vi "Lockin Digitizer Output Signal.vi"(6 "decimating factor":i32=1, 8 "error in":errorcluster, 9 "Phase in":dbl format="%0.2f", 10 "Frequency":dbl=0.0078125 format="%0.4e", 11 "Input data":dbl[][](array[numeric])) -> (0 "error out":errorcluster, 1 "Phase out":dbl format="%0.2e", 2 "Y":dbl[][](array[numeric]), 3 "X":dbl[][](array[numeric]))   [LabVIEW 2021]
uses:
  <vilib>/Analysis/2dsp.llb/Decimate (single shot, DBL).vi
  <vilib>/Analysis/NI_AALBase.lvlib
  <vilib>/Analysis/NI_AALPro.lvlib
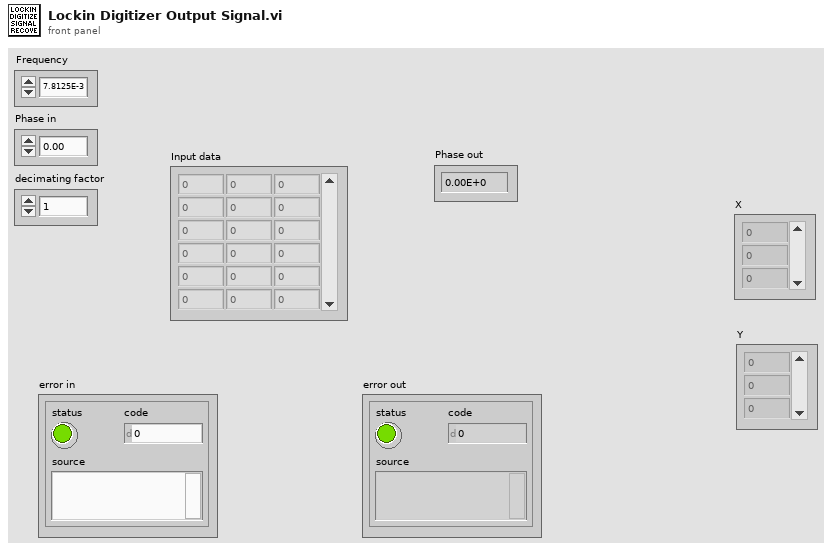
[diagram p1: front panel]
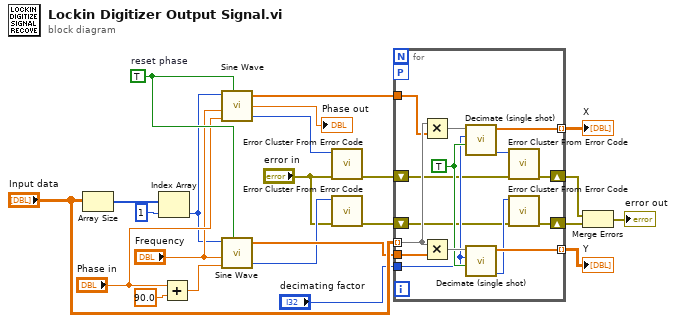
[diagram p0: block diagram]
diagram:
  w17 = TRUE  # reset phase
  n1 = Array Size(array="Input data") -> (size(s)=w23:i32[])
  n2 = Index Array(array=w23, index=1) -> (element=w12:i32)
  n3 = Add(x="Phase in", y=90.0 ("phase in")) -> (x+y=w14:dbl)
  n4 = call <vilib>:"Sine Wave.vi"("samples"=w12, "frequency"="Frequency", "phase in"="Phase in", "reset phase"=w17) -> ("sine wave"=w18:dbl[], "phase out"=→"Phase out":dbl, "error"=w20:i32)  [unwired: 1 in]
  n5 = call <vilib>:"Sine Wave.vi"("samples"=w12, "frequency"="Frequency", "phase in"=w14, "reset phase"=w17) -> ("sine wave"=w11:dbl[], "error"=w9:i32)  [unwired: 1 in, 1 out]
  n6 = call <vilib>:"Error Cluster From Error Code.vi"("error in (no error)"="error in", "error code (0)"=w20) -> ("error out"=w8:errorcluster)  [unwired: 7 in]
  n7 = call <vilib>:"Error Cluster From Error Code.vi"("error in (no error)"="error in", "error code (0)"=w9) -> ("error out"=w7:errorcluster)  [unwired: 7 in]
  n8 = for {
    tunnel: "Input data" -> [w38] mode=indexing
    tunnel: w18 -> [w37]
    tunnel: w11 -> [w33]
    workers-P: _ -> [_]
    tunnel: "decimating factor" -> [w32]
    tunnel: [w31] -> w4 mode=indexing
    tunnel: [w30] -> w3 mode=indexing
    shift-right: [w26] -> w6
    shift-left: w8 -> [w27]
    shift-right: [w24] -> w5
    shift-left: w7 -> [w25]
    w34 = TRUE ("averaging")
    n9 = Multiply(x=w38, y=w37) -> (x*y=w35:dbl[])
    n10 = Multiply(x=w38, y=w33) -> (x*y=w36:dbl[])
    n11 = call-poly <vilib>:"Decimate (single shot).vi"("averaging"=w34, "decimating factor"=w32, "X"=w35) -> ("error"=w29:i32, "Decimated Array"=w31:dbl[])  [unwired: 7 in]
    n12 = call-poly <vilib>:"Decimate (single shot).vi"("averaging"=w34, "decimating factor"=w32, "X"=w36) -> ("error"=w28:i32, "Decimated Array"=w30:dbl[])  [unwired: 7 in]
    n13 = call <vilib>:"Error Cluster From Error Code.vi"("error in (no error)"=w27, "error code (0)"=w29) -> ("error out"=w26:errorcluster)  [unwired: 7 in]
    n14 = call <vilib>:"Error Cluster From Error Code.vi"("error in (no error)"=w25, "error code (0)"=w28) -> ("error out"=w24:errorcluster)  [unwired: 7 in]
  }
  "Y" <- w3
  "X" <- w4
  n15 = Merge Errors(w6, w5) -> (→"error out":errorcluster)
